vi "Read Field Type.vi"(7 "field name":string, 8 "error in (no error)":errorcluster, 11 "Value in":refnum<class "Value.lvclass">) -> (0 "error out":errorcluster, 2 "type code":T1, 3 "Value out":refnum<class "Value.lvclass">)   [LabVIEW 2020, in "Value.lvlib" / "Value.lvclass"]
uses:
  Value.lvclass
  Value.lvclass/Value.ctl
  Type Code.ctl
  Value.lvlib
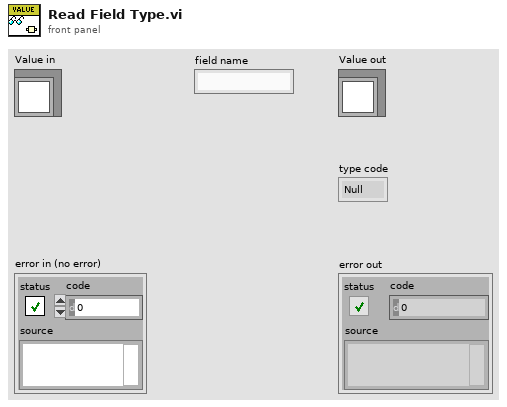
[diagram p1: front panel]
types:
  T1 = typedef "Value.lvlib/Type Code.ctl" = enum8{"Null", "Bool", "BoolA", "Int8", "Int8A", "Int16", "Int16A", "Int32", "Int32A", "Int64", "Int64A", "UInt8", "UInt8A", "UInt16", "UInt16A", "UInt32", "UInt32A", "UInt64", "UInt64A", "Float32", "Float32A", "Float64", "Float64A", "String", "StringA", "Struct", "StructA", "Union", "UnionA", "Any", "AnyA"}
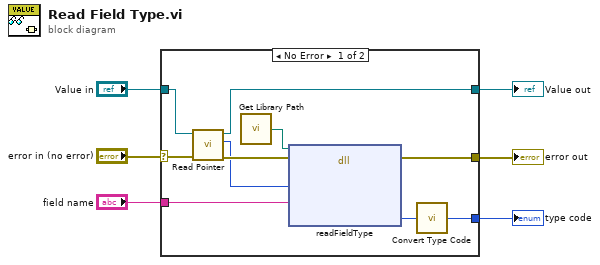
[diagram p0: block diagram]
diagram:
  n1 = case shown="No Error" "error in (no error)" {
    selector: "error in (no error)" -> [w15 w18]
    tunnel: [w16 w18] -> w5
    tunnel: "Value in" -> [w12 w17]
    tunnel: [w9 w17] -> w3
    tunnel: "field name" -> [w10 _]
    tunnel: [w8 _] -> w1
    frame No Error {
      n2 = call-dynamic "Read Pointer.vi"("error in (no error)"=w15, "Value in"=w12) -> ("error out"=w14:errorcluster, "pointer"=w11:i64, "Value out"=w9:refnum<class "Value.lvclass">)  [unwired: 7 in]
      n3 = call "Get Library Path.vi"() -> ("Path"=w13:path)  [unwired: 1 in]
      n4 = dll-call lib="?" fn="readFieldType"(path in=w13, error in=w14, "value"=w11, "field_name"=w10) -> (error out=w16:errorcluster, "type_code"=w7:u8)  [unwired: 5 in, 1 out]
      n5 = call "Convert Type Code.vi"("pvxs type code"=w7) -> ("type code"=w8:T1)
    }
    frame Error {
    }
  }
  "error out" <- w5
  "Value out" <- w3
  "type code" <- w1
